vi "get_chessboard_square.vi"(1 "column":u8, 2 "row":u8, 3 "chessboard":T1[][](array[typedef])) -> (0 "chessboard_square":T1)   [LabVIEW 2020, in "core.lvlib"]
uses:
  core.lvlib
  core_data/chess_square.ctl
  core_data/neighbour_square.ctl
  core_data/core_data.lvlib
panel:
  # "Development\ncontrols/indicators useful for development and testing, but which are not outputs of the VI"
  # "Input\nInputs to the VI"
  # "Output\nOutputs of the VI"
  # "Description\n\nBlank VI with error handling case. \n\nSummarize the use of this VI in this space."
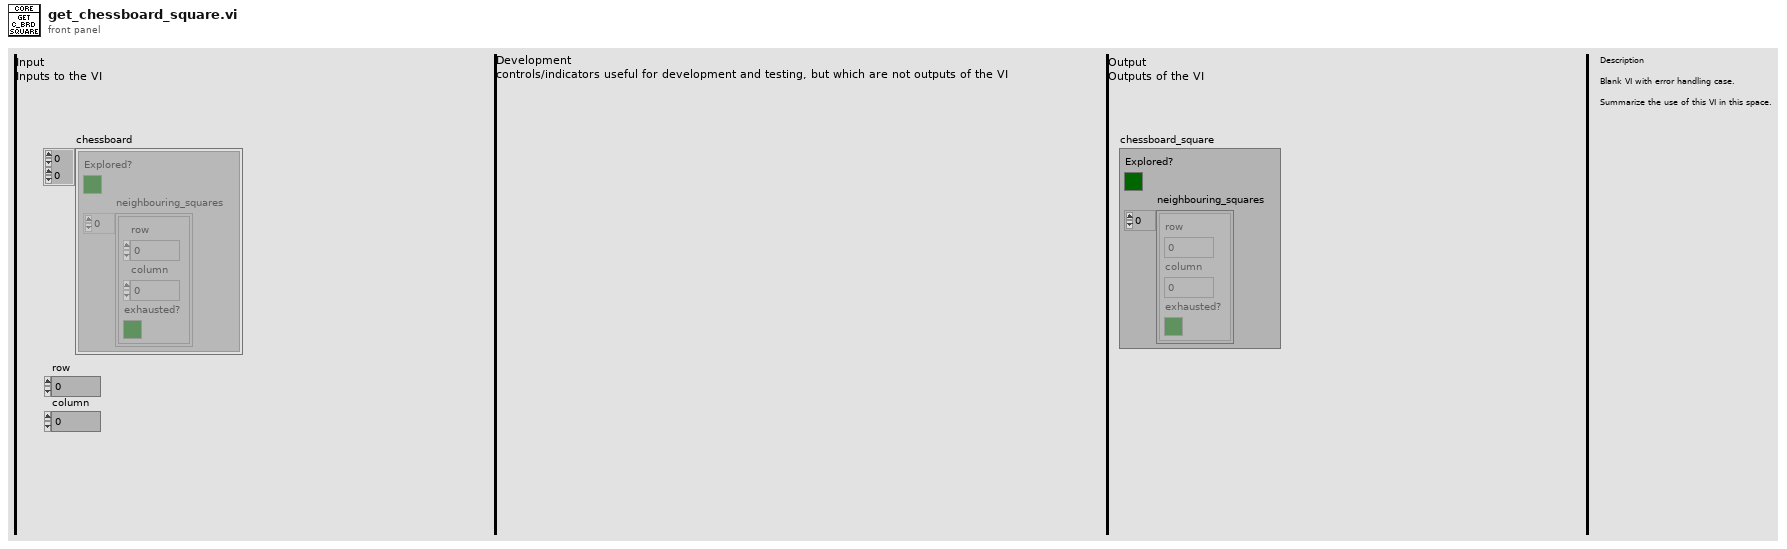
[diagram p1: front panel]
types:
  T1 = typedef "core.lvlib/core_data.lvlib/chess_square.ctl" = cluster{"Explored?":bool, "neighbouring_squares":T2[]}
  T2 = typedef "core.lvlib/core_data.lvlib/neighbour_square.ctl" = cluster{"row":u8, "column":u8, "exhausted?":bool}
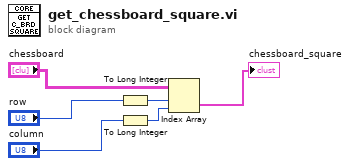
[diagram p0: block diagram]
diagram:
  n1 = To Long Integer(number="row") -> (32bit integer=w4:i32)
  n2 = To Long Integer(number="column") -> (32bit integer=w3:i32)
  n3 = Index Array(array="chessboard", index (row)=w4, index (col)=w3) -> (element=→"chessboard_square":T1)
